vi "Triggered Test Logger.vi"() -> ()   [LabVIEW 2013]
doc: "Recommended Input Signal: 10 Hz, 1.8 Vpp, sine wave\n\nThis example requires NI-Scope 3.3 or later.\nDevices Supported: NI 5112, NI 5620, NI 5621, NI 5122, NI 5124, NI 5922, NI 5114, NI 5142\n\nVI Description:\n\nThis example demonstrates using continuous acquisition to fetch a user-defined, but quite large record of data all while continuously streaming the data to a binary file using the Win32 File I/O VIs. The digitizer is configured using the Configure Vertical and Configure Horizontal VI's. Auto setup in this case may not be useful, as it may choose a horizontal rate that exceeds the computer's streaming capabilities.\n\nIn this example, continuous acquisition is used. This allows the user to start the digitizer, and continuously fetch data without losing any points. This is accomplished by configuring a software trigger and never sending the software trigger. Therefore, the digitizer will continuously acquire data into its onboard memory until Abort or Close is called.\n\nThe producer loop continuously fetches data from onboard memory into the LabVIEW memory using DMA transfers. This data is placed into a queue in order to efficiently transfer the data to a parallel consumer loop where it is written file. If the sampling rate is low, the computer can fetch all the data from the digitizer, so data is never overwritten. However, at faster sampling rates, the computer will not be able to fetch the data before it is overwritten by new data. This results in the \"data overwritten\" error.\n\nThe consumer loop continuously empties data from the queue and writes data to disk using the Win32 Write File.vi. The file is opened using the Win32 Open File.vi, which disables Windows caching during the write process, resulting in increased performance. However when Windows caching is disabled, <b>data must be written to file in a multiple of the sector size of the disk (typically 512 bytes).</b>"
uses:
  <vilib>/Utility/error.llb/DialogType.ctl
  <vilib>/Waveform/WDTFileIO.llb/ Write Waveforms to File (1D).vi
  Breakdown Acoustics Controls.lvlib
panel:
  out "# DAQ Restarts":i32
  out "# Triggers":i32
  in  "Tab Control":T1(tab)
  in  "Max Queue Size":i32=8
  in  "Samples Per Channel":i32=5120 caption="Max Points Per Fetch" step=1048576
  in  "Configuration File":path=path "C:/Users/plane/Dropbox/Research/MTA/DAQ VIs/Breakdown Acoustics Controls/MC_test.xml"
  in  "Sample Rate":i32=100000
  in  "Queue Timeout (ms)":i32=100
  out "Data Directory":path
  in  "Reset Raw Signals Graph":bool
  out "Raw Signals":waveform(dbl)[](graph)
  out "# Microphones":i32
  in  "stop":bool
  out "Acquisition Status":bool
  # "Configuration Settings"
  # "Acquisition Settings"
  # "(should be a multiple of disk sector size)"
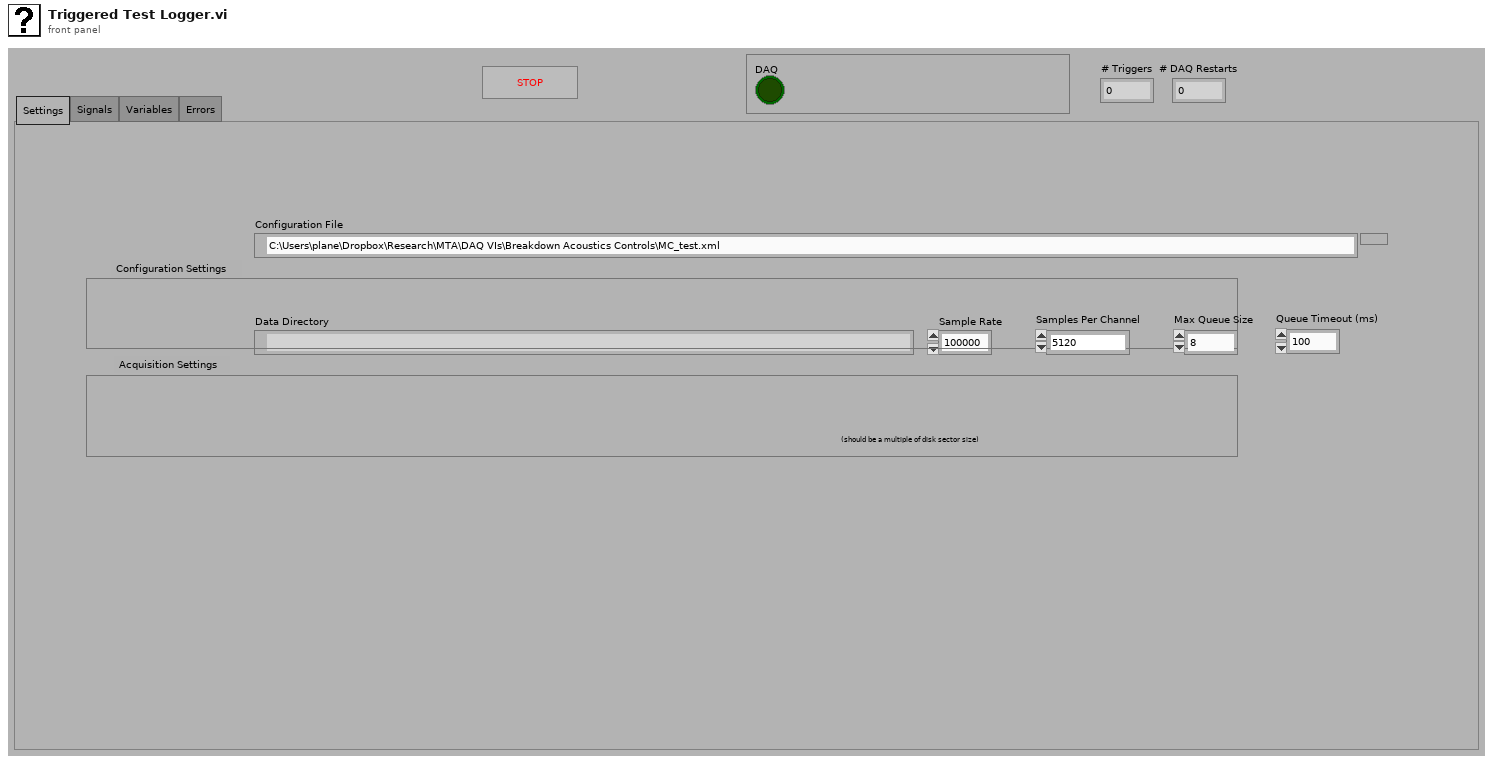
[diagram p1: front panel]
types:
  T1 = enum32{"Settings", "Signals", "Variables", "Errors"}
  T2 = typedef "DialogType.ctl" = u16
  T3 = cluster{"X Scale.Range:Minimum":dbl, "Y Scale.Range:Minimum":dbl, "X Scale.Range:Maximum":dbl, "Y Scale.Range:Maximum":dbl}
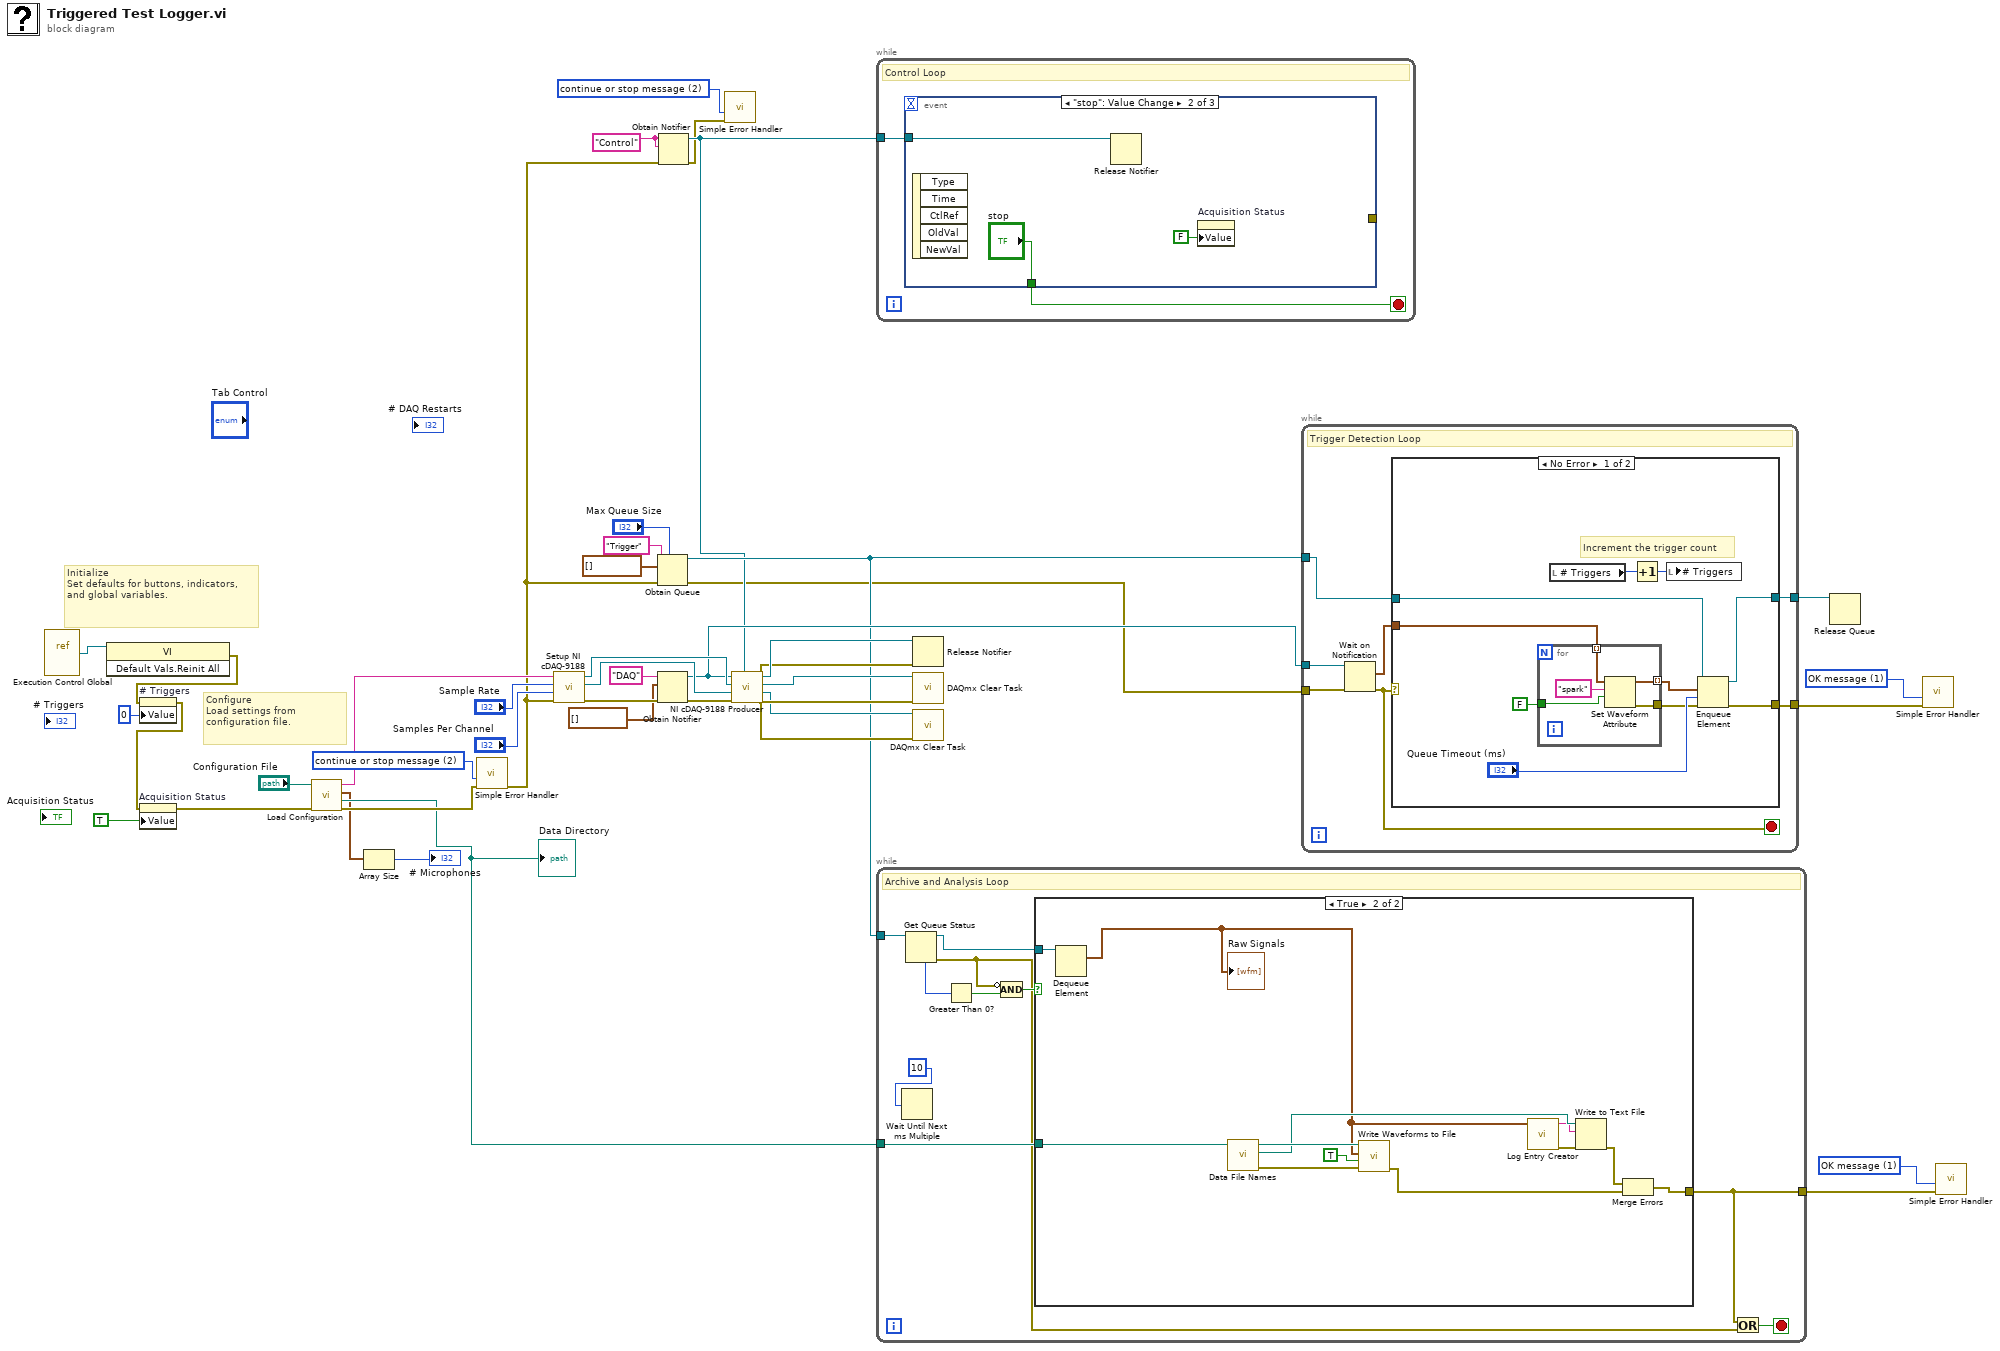
[diagram p0: block diagram]
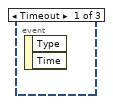
[diagram p3: hidden frame]
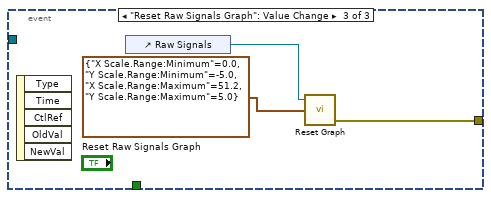
[diagram p4: hidden frame]
diagram:
  w2 = T2 1 items=["no dialog", "OK message", "continue or stop message", "OK message + warnings", "continue/stop + warnings"] ("type of dialog (OK msg:1)")
  w5 = T2 1 items=["no dialog", "OK message", "continue or stop message", "OK message + warnings", "continue/stop + warnings"] ("type of dialog (OK msg:1)")
  w9 = T2 2 items=["no dialog", "OK message", "continue or stop message", "OK message + warnings", "continue/stop + warnings"] ("type of dialog (OK msg:1)")
  w22 = "Control" ("name (unnamed)")
  w40 = T2 2 items=["no dialog", "OK message", "continue or stop message", "OK message + warnings", "continue/stop + warnings"] ("type of dialog (OK msg:1)")
  # "Configure\nLoad settings from configuration file."
  # "Initialize\nSet defaults for buttons, indicators, and global variables."
  n1 = vi-ref "Execution Control Global.vi"() -> (w35:refnum<vi>)
  n2 = invoke class="VI" method="Default Vals.Reinit All"(reference=w35) -> (error out=w34:errorcluster)  [unwired: 2 in, 2 out]
  n3 = property on="# Triggers" class="DigNum (strict)"(error in=w34, "Value"=0 ("# Triggers")) -> (error out=w13:errorcluster)  [unwired: 1 in, 1 out]
  n4 = property on="Acquisition Status" class="Bool (strict)"(error in=w13, "Value"=TRUE ("Acquisition Status")) -> (error out=w36:errorcluster)  [unwired: 1 in, 1 out]
  n5 = call "Load Configuration.vi"("error in"=w36, "Configuration File"="Configuration File") -> ("error out"=w21:errorcluster, "Data Directory"=w4:path, "Microphone Locations"=w1:cluster{"r":dbl, "theta":dbl, "z":dbl}[], "DAQ Channels"=w31:string)  [unwired: 6 in]
  "Data Directory" <- w4
  n6 = Array Size(array=w1) -> (size(s)=→"# Microphones":i32)
  n7 = call <vilib>:"Simple Error Handler.vi"("type of dialog (OK msg:1)"=w40, "error in (no error)"=w21) -> ("error out"=w18:errorcluster)  [unwired: 3 in, 4 out]
  n8 = call "Setup NI cDAQ-9188.vi"("error in"=w18, "Samples per Channel"="Samples Per Channel", "Sample Rate"="Sample Rate", "Physical Channels"=w31) -> ("error out"=w28:errorcluster, "Counter Task"=w25:refnum<k21>, "AI Voltage Task"=w24:refnum<k21>)  [unwired: 5 in]
  n9 = Obtain Queue(max queue size (-1, unlimited)="Max Queue Size", name (unnamed)="Trigger", element data type=waveform(dbl)[] [], error in (no error)=w18) -> (queue out=w12:refnum<queue>, error out=w10:errorcluster)  [unwired: 1 in, 1 out]
  n10 = Obtain Notifier(name (unnamed)="DAQ", notification data type=waveform(dbl)[] [] ("data"), error in (no error)=w28) -> (notifier out=w20:refnum<notifier>, error out=w26:errorcluster)  [unwired: 1 in, 1 out]
  n11 = Obtain Notifier(name (unnamed)=w22, notification data type=w22, error in (no error)=w18) -> (notifier out=w11:refnum<notifier>, error out=w8:errorcluster)  [unwired: 1 in, 1 out]
  n12 = call <vilib>:"Simple Error Handler.vi"("type of dialog (OK msg:1)"=w9, "error in (no error)"=w8) -> ()  [unwired: 3 in, 5 out]
  n13 = call "NI cDAQ-9188 Producer.vi"("Control Notifier"=w11, "error in"=w26, "Counter Task"=w25, "AI Voltage Task"=w24, "DAQ Notifier"=w20) -> ("error out"=w15:errorcluster, "Counter Task out"=w14:refnum<k21>, "AI Voltage Task out"=w16:refnum<k21>, "DAQ Notifier out"=w17:refnum<notifier>)  [unwired: 3 in]
  n14 = while {
    tunnel: w11 -> [w42]
    stop <- w43 stop-if-true
    # "Control Loop"
    n15 = event shown="[1] \"stop\": Value Change" {
      selector: _ -> [_ _ _]
      dyn-events: _ -> [_ _ _]
      timeout: _ -> [_ _ _]
      tunnel: [_ _ w47] -> _
      tunnel: [_ "stop" _] -> w43
      tunnel: w42 -> [_ w45 _]
      event Timeout {
        n16 = event-data() -> ()  [unwired: 1 in, 2 out]
      }
      event "stop": Value Change {
        n17 = event-data() -> ()  [unwired: 1 in, 5 out]
        n18 = Release Notifier(notifier=w45) -> ()  [unwired: 2 in, 3 out]
        n19 = property on="Acquisition Status" class="Bool (strict)"("Value"=FALSE ("Acquisition Status")) -> ()  [unwired: 2 in, 2 out]
      }
      event "Reset Raw Signals Graph": Value Change {
        n20 = event-data() -> ()  [unwired: 1 in, 5 out]
        n21 = control-ref of="Raw Signals"() -> (w49:refnum<vi>)
        n22 = call "Reset Graph.vi"("Graph Boundaries"=T3 {"X Scale.Range:Minimum"=0.0, "Y Scale.Range:Minimum"=-5.0, "X Scale.Range:Maximum"=51.2, "Y Scale.Range:Maximum"=5.0}, "Graph Reference"=w49) -> ("error out"=w47:errorcluster)  [unwired: 3 in]
      }
    }
  }
  n23 = while {
    tunnel: w12 -> [w59]
    tunnel: w4 -> [w55]
    tunnel: [w50] -> w3
    stop <- w52 stop-if-true
    # "Archive and Analysis Loop"
    n24 = Wait Until Next ms Multiple(millisecond multiple=u32 10) -> ()  [unwired: 1 out]
    n25 = Get Queue Status(queue=w59) -> (queue out=w57:refnum<queue>, error out=w51:errorcluster, # elements in queue=w58:i32)  [unwired: 2 in, 5 out]
    n26 = Greater Than 0?(x=w58) -> (x > 0?=w54:bool)
    n27 = Compound Arithmetic op=AND(invert w51, w54) -> (w53:bool)
    n28 = case shown="True" w53 {
      tunnel: w57 -> [_ w71]
      tunnel: w55 -> [_ w69]
      tunnel: [_ w65] -> w50
      frame False {
      }
      frame True {
        n29 = Dequeue Element(queue=w71) -> (element=w60:waveform(dbl)[])  [unwired: 2 in, 3 out]
        "Raw Signals" <- w60
        n30 = call "Data File Names.vi"("Data Directory"=w69) -> ("error out"=w67:errorcluster, "Log File"=w64:path, "Raw Data File"=w68:path)  [unwired: 7 in, 1 out]
        n31 = call-poly <vilib>:"Write Waveforms to File.vi"("error in (no error)"=w67, "append to file? (new file:F)"=TRUE, "waveform array"=w60, "file path (dialog if empty)"=w68) -> ("error out"=w66:errorcluster)  [unwired: 6 in, 1 out]
        n32 = call "Log Entry Creator.vi"("Waveforms"=w60) -> ("error out"=w62:errorcluster, "Log Entry"=w63:string)  [unwired: 9 in]
        n33 = Write to Text File(file (use dialog)=w64, text=w63, error in=w62) -> (error out=w61:errorcluster)  [unwired: 1 in, 2 out]
        n34 = Merge Errors(w61, w66) -> (w65:errorcluster)
      }
    }
    n35 = Or(x=w50, y=w51) -> (x .or. y?=w52:bool)
  }
  n36 = Release Notifier(notifier=w17, error in (no error)=w15) -> ()  [unwired: 1 in, 3 out]
  n37 = call <vilib>:"DAQmx Clear Task.vi"("task in"=w16, "error in"=w15) -> ()  [unwired: 13 in, 1 out]
  n38 = call <vilib>:"DAQmx Clear Task.vi"("task in"=w14, "error in"=w15) -> ()  [unwired: 13 in, 1 out]
  n39 = while {
    tunnel: w20 -> [w78]
    tunnel: w10 -> [w76]
    tunnel: w12 -> [w75]
    tunnel: [w73] -> w6
    tunnel: [w72] -> w7
    stop <- w77 stop-if-true
    # "Trigger Detection Loop"
    n40 = Wait on Notification(notifier=w78, error in (no error)=w76) -> (notification=w74:waveform(dbl)[], error out=w77:errorcluster)  [unwired: 4 out]
    n41 = case shown="No Error" w77 {
      selector: w77 -> [_ w94]
      tunnel: w75 -> [w88 w95]
      tunnel: w74 -> [w80 _]
      tunnel: [w86 w94] -> w73
      tunnel: [w85 w95] -> w72
      frame No Error {
        # "Increment the trigger count"
        n42 = for {
          tunnel: w80 -> [w92] mode=indexing
          tunnel: [w91] -> w82 mode=indexing
          tunnel: [w90] -> w81
          tunnel: FALSE ("Spark!") -> [w89]
          n43 = Set Waveform Attribute(5:w89, 6:"spark" ("name"), 7:w92) -> (0:w90:errorcluster, 3:w91:waveform(dbl))  [unwired: 1 in, 1 out]
        }
        n44 = local read "# Triggers"() -> (w83:i32)
        n45 = Increment(x=w83) -> (x+1=w84:i32)
        n46 = local write "# Triggers"(w84) -> ()
        n47 = Enqueue Element(queue=w88, element=w82, timeout in ms (-1)="Queue Timeout (ms)", error in (no error)=w81) -> (queue out=w85:refnum<queue>, error out=w86:errorcluster)  [unwired: 1 out]
      }
      frame Error {
      }
    }
  }
  n48 = Release Queue(queue=w7) -> ()  [unwired: 2 in, 3 out]
  n49 = call <vilib>:"Simple Error Handler.vi"("type of dialog (OK msg:1)"=w5, "error in (no error)"=w6) -> ()  [unwired: 3 in, 5 out]
  n50 = call <vilib>:"Simple Error Handler.vi"("type of dialog (OK msg:1)"=w2, "error in (no error)"=w3) -> ()  [unwired: 3 in, 5 out]
